vi "transpose_2D_array.vi"(10 "Image Pixels (U8) in":u8[][](array[numeric]), 11 "flip direction":bool) -> (3 "Image Pixels (U8) out":u8[][](array[numeric]))   [LabVIEW 2011]
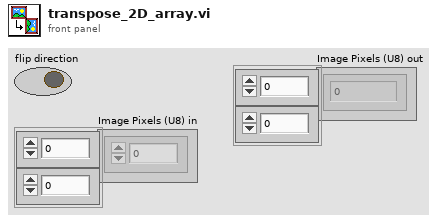
[diagram p1: front panel]
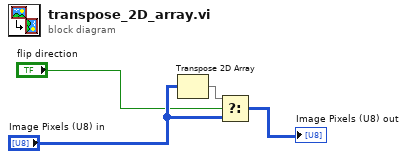
[diagram p0: block diagram]
diagram:
  n1 = Transpose 2D Array(2D array="Image Pixels (U8) in") -> (transposed array=w3:u8[][])
  n2 = Select(t=w3, s="flip direction", f="Image Pixels (U8) in") -> (s? t:f=→"Image Pixels (U8) out":u8[][])
